vi "Read Input FIFO.vi"(8 "error in (no error)":errorcluster, 11 "Engine Run Time Data in":T1) -> (0 "error out":errorcluster, 3 "Engine Run Time Data out":T1)   [LabVIEW 2017]
uses:
  Controls/Channel Mode.ctl
  NI 272x Resistive Simulation Custom Device Shared.lvlib
  <instrlib>/ni272xReferenceVIs/ni272xReferenceVIs.llb/ni272x Callendar-Van Dusen RTD Parameters.ctl
  Controls/Compiled HW Channel.ctl
  Controls/Compiled Connect Channel.ctl
  Controls/Compiled Engine Data.ctl
  <instrlib>/ni272xReferenceVIs/ni272xReferenceVIs.llb/ni272x Reference.ctl
  Controls/Engine Run Time Data.ctl
  NI 272x Resistive Simulation Custom Device Engine.lvlib
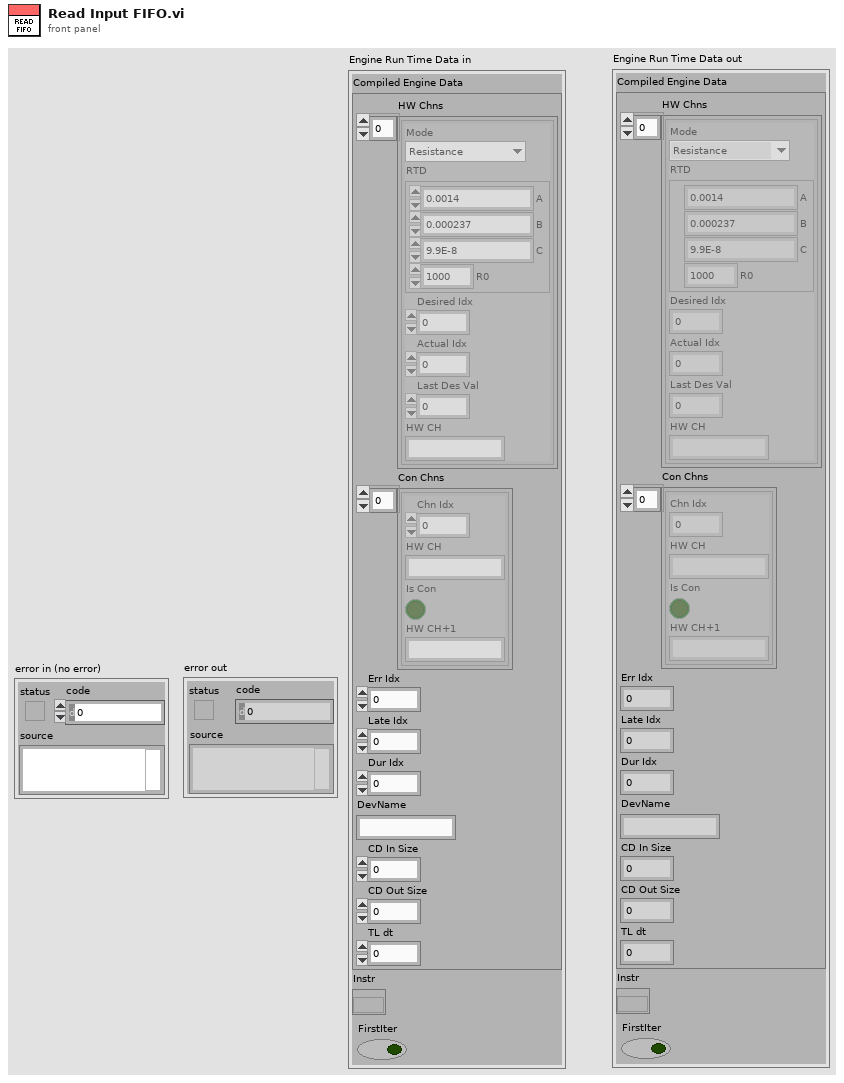
[diagram p1: front panel]
types:
  T1 = typedef "NI 272x Resistive Simulation Custom Device Engine.lvlib/Engine Run Time Data.ctl" = cluster{"Compiled Engine Data":T2, "Instr":T7, "FirstIter":bool}
  T2 = typedef "NI 272x Resistive Simulation Custom Device Shared.lvlib/Compiled Engine Data.ctl" = cluster{"HW Chns":T3[], "Con Chns":T6[], "Err Idx":i32, "Late Idx":i32, "Dur Idx":i32, "DevName":string, "CD In Size":i32, "CD Out Size":i32, "TL dt":i64}
  T3 = typedef "NI 272x Resistive Simulation Custom Device Shared.lvlib/Compiled HW Channel.ctl" = cluster{"Mode":T4, "RTD":T5, "Desired Idx":i32, "Actual Idx":i32, "Last Des Val":dbl, "HW CH":string}
  T4 = typedef "NI 272x Resistive Simulation Custom Device Shared.lvlib/Channel Mode.ctl" = enum16{"Resistance", "RTD Temperature"}
  T5 = typedef "ni272x Callendar-Van Dusen RTD Parameters.ctl" = cluster{"A":dbl, "B":dbl, "C":dbl, "R0":dbl}
  T6 = typedef "NI 272x Resistive Simulation Custom Device Shared.lvlib/Compiled Connect Channel.ctl" = cluster{"Chn Idx":i32, "HW CH":string, "Is Con":bool, "HW CH+1":string}
  T7 = typedef "ni272x Reference.ctl" = refnum<k20>
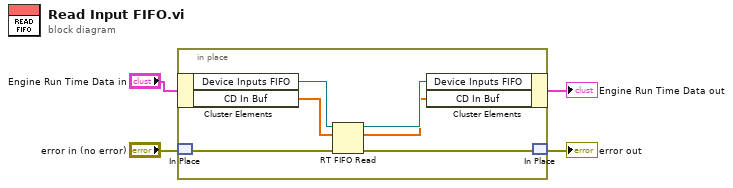
[diagram p0: block diagram]
diagram:
  n1 = in-place {
    n2 = in-place-cluster #1("Engine Run Time Data in") -> ("Device Inputs FIFO"=w8:refnum<k33>, "CD In Buf"=w9:dbl[])
    n3 = in-place-match #2("error in (no error)") -> (w10:errorcluster)
    n4 = RT FIFO Read(0:w8, 1:w9, 3:w10) -> (8:w7:refnum<k33>, 9:w6:dbl[], 11:w5:errorcluster)  [unwired: 1 in, 2 out]
    n5 = in-place-cluster #1("Device Inputs FIFO"=w7, "CD In Buf"=w6) -> (→"Engine Run Time Data out":T1)
    n6 = in-place-match #2(w5) -> (→"error out":errorcluster)
  }
